vi "Image_Viewer_main.vi"() -> ()   [LabVIEW 2020]
uses:
  #typedef_Program_Data.ctl
  <vilib>/Utility/miscctls.llb/LVBoundsTypeDef.ctl
  <vilib>/event_ctls.llb/eventvkey.ctl
panel:
  out "Program Data":T1
  out "new picture":picture
  out "Multi Listbox":i32(listbox)=-1
  in  "Path":path
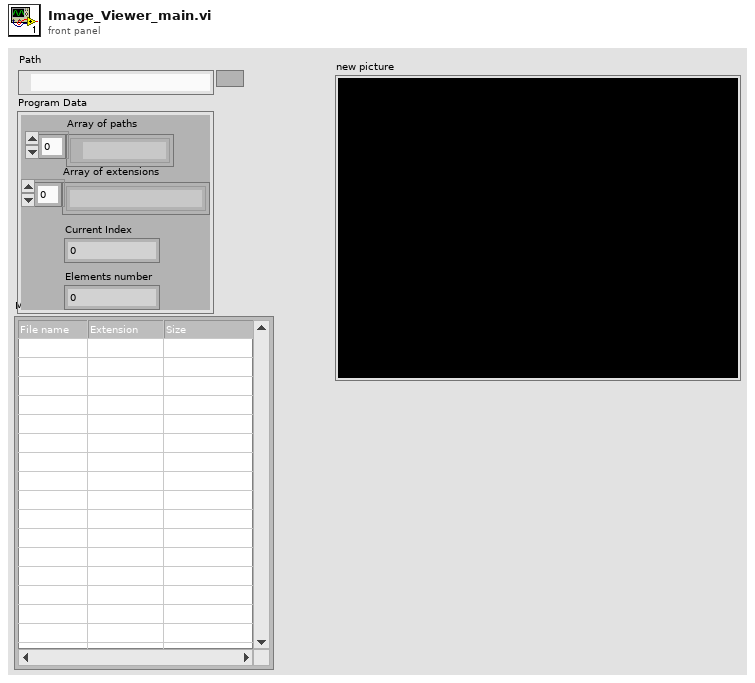
[diagram p1: front panel]
types:
  T1 = typedef "#typedef_Program_Data.ctl" = cluster{"Array of extensions ":string[], "Array of paths":path[], "Current Index":i32, "Elements number":i32}
  T2 = typedef "LVBoundsTypeDef.ctl" = cluster{"Width":u32, "Height":u32}
  T3 = typedef "imagedata.ctl" = cluster{"image type":i32, "image depth":i32, "image":u8[], "mask":u8[], "colors":u32[], "Rectangle":cluster{"left":i16, "top":i16, "right":i16, "bottom":i16}}
  T4 = typedef "eventvkey.ctl" = enum16{"ASCII", "Enter", "Return", "Shift", "Ctrl", "Alt", "Cmd", "Opt", "Caps", "NumLock", "Clear", "Break", "Up", "Down", "Left", "Right", "Insert", "Delete", "Home", "End", "PageUp", "PageDown", "Escape", "Help", "Pause", "ScrollLock", "F1", "F2", "F3", "F4", "F5", "F6", "F7", "F8", "F9", "F10", "F11", "F12", "F13", "F14", "F15", "F16", "F17", "F18", "F19", "F20", "F21", "F22", "F23", "F24", "Play", "VolumeUp", "VolumeDown", "Mute", "Two Byte Char"}
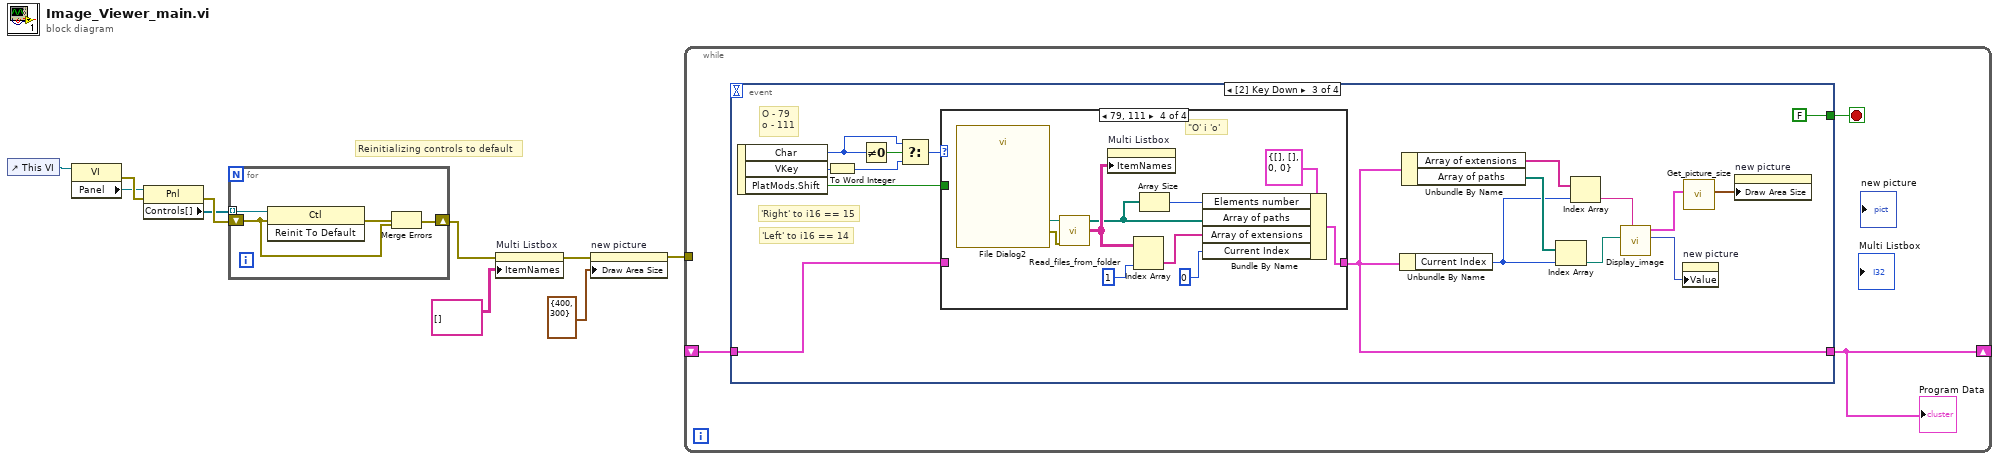
[diagram p0: block diagram]
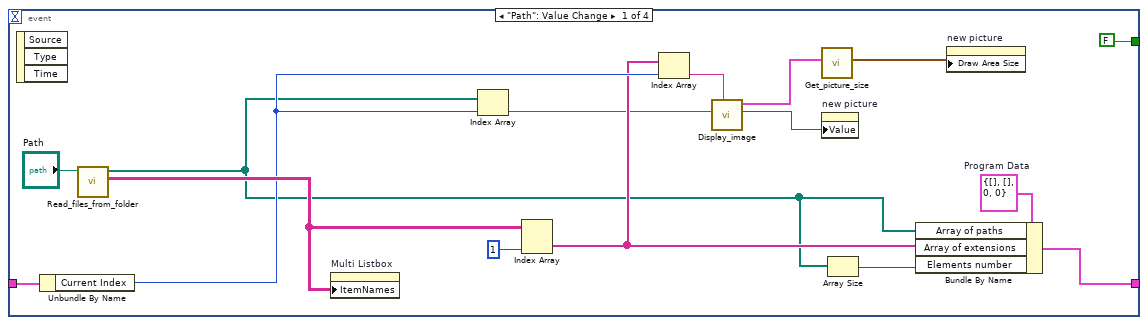
[diagram p2: hidden frame]
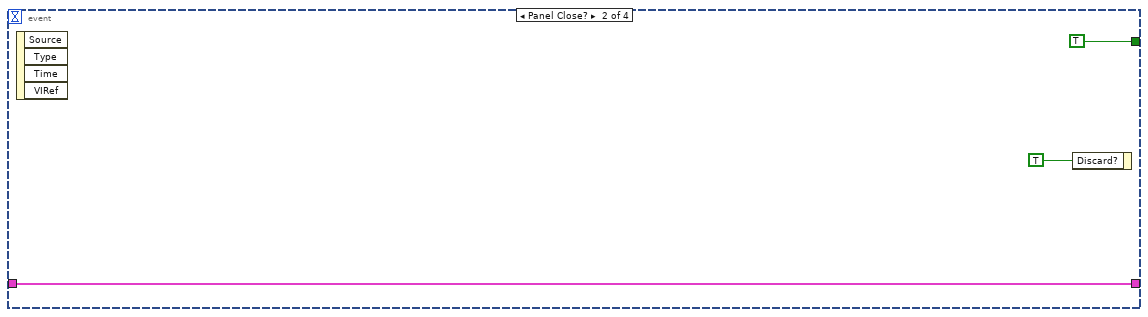
[diagram p3: hidden frame]
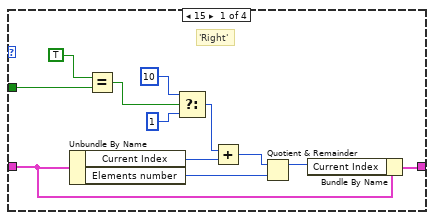
[diagram p4: hidden frame]
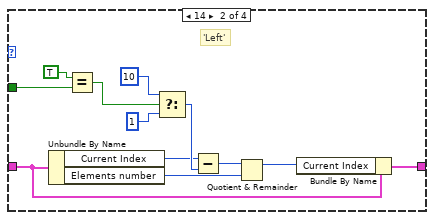
[diagram p5: hidden frame]
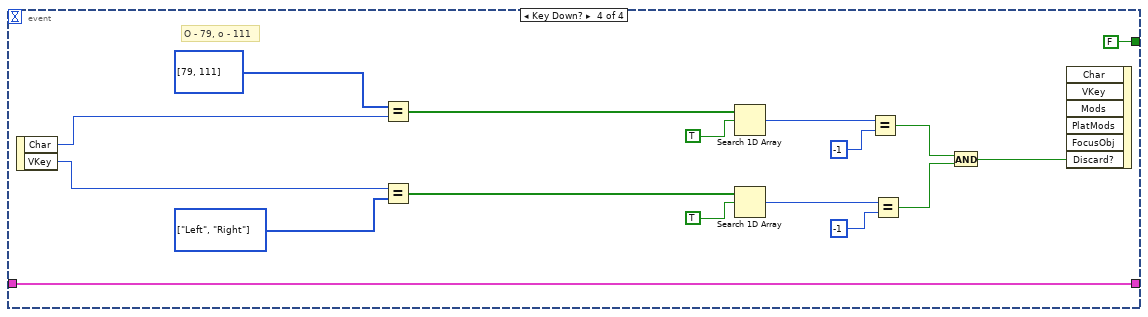
[diagram p7: hidden frame]
diagram:
  # "Reinitializing controls to default"
  n1 = control-ref of="This VI"() -> (w5:refnum<vi>)
  n2 = property class="VI"(reference=w5) -> (error out=w8:errorcluster, "Panel"=w6:refnum<vi>)  [unwired: 1 in, 1 out]
  n3 = property class="Pnl"(reference=w6, error in=w8) -> (error out=w9:errorcluster, "Controls[]"=w7:refnum<vi>[])  [unwired: 1 out]
  n4 = for {
    tunnel: w7 -> [w14] mode=indexing
    shift-right: [w13] -> w2
    shift-left: w9 -> [w12]
    n5 = invoke class="Ctl" method="Reinit To Default"(reference=w14, error in=w12) -> (error out=w11:errorcluster)  [unwired: 1 in, 2 out]
    n6 = Merge Errors(w11, w12) -> (w13:errorcluster)
  }
  n7 = property on="Multi Listbox" class="MCListbox (strict)"(error in=w2, "ItemNames"=string[][] [] ("Item Names")) -> (error out=w1:errorcluster)  [unwired: 1 in, 1 out]
  n8 = property on="new picture" class="Pict"(error in=w1, "Draw Area Size"=T2 {"Width"=400, "Height"=300}) -> (error out=w10:errorcluster)  [unwired: 1 in, 1 out]
  n9 = while {
    shift-right: [w16] -> _
    shift-left: _ -> [w17]
    tunnel: w10 -> [_]
    stop <- w15 stop-if-true
    n10 = event shown="[2] Key Down" {
      selector: _ -> [_ _ _ _]
      dyn-events: _ -> [_ _ _ _]
      timeout: _ -> [_ _ _ _]
      tunnel: w17 -> [w29 w34 w40 w99]
      tunnel: [w18 w34 w38 w99] -> w16
      tunnel: [FALSE TRUE FALSE FALSE] -> w15
      event "Path": Value Change {
        w31 = T1 {"Array of extensions "=[], "Array of paths"=[], "Current Index"=0, "Elements number"=0}  # Program Data
        n11 = event-data() -> ()  [unwired: 1 in, 3 out]
        n12 = Unbundle By Name(w29) -> ("Current Index"=w28:i32)
        n13 = call "Read_files_from_folder.vi"("Path"="Path") -> ("Array of strings (file name, extension, size (in bytes))"=w33:string[][], "File Path"=w20:path[])  [unwired: 8 in, 1 out]
        n14 = property on="Multi Listbox" class="MCListbox (strict)"("ItemNames"=w33) -> ()  [unwired: 2 in, 2 out]
        n15 = Index Array(array=w20, index=w28) -> (element=w26:path)
        n16 = Index Array(array=w33, index (col)=1 ("disabled index (col)")) -> (element=w27:string[])  [unwired: 1 in]
        n17 = Index Array(array=w27, index=w28) -> (element=w24:string)
        n18 = call "Display_image.vi"("lowercase file extension"=w24, "path file"=w26) -> ("picture"=w25:picture, "image data"=w22:T3)  [unwired: 7 in, 1 out]
        n19 = call "Get_picture_size.vi"("image data"=w22) -> ("Draw Area Size"=w21:T2)  [unwired: 9 in, 1 out]
        n20 = property on="new picture" class="Pict"("Value"=w25) -> ()  [unwired: 2 in, 2 out]
        n21 = Array Size(array=w20) -> (size(s)=w19:i32)
        n22 = Bundle By Name(cluster=w31, "Array of paths"=w20, "Array of extensions"=w27, "Elements number"=w19) -> (w18:T1)
        n23 = property on="new picture" class="Pict"("Draw Area Size"=w21) -> ()  [unwired: 2 in, 2 out]
      }
      event Panel Close? {
        n24 = event-data() -> ()  [unwired: 1 in, 4 out]
        n25 = event-data("Discard?"=TRUE) -> ()  [unwired: 1 in, 1 out]
      }
      event Key Down {
        # "O - 79\no - 111"
        # "'Left' to i16 == 14"
        # "'Right' to i16 == 15"
        n26 = event-data() -> ("Char"=w44:i16, "VKey"=w43:T4, "PlatMods.Shift"=w39:bool)  [unwired: 1 in]
        n27 = To Word Integer(number=w43) -> (16bit integer=w42:i16)
        n28 = Not Equal To 0?(x=w44) -> (x != 0?=w45:bool)
        n29 = Select(t=w44, s=w45, f=w42) -> (s? t:f=w41:i16)
        n30 = case shown="79, 111" w41 {
          tunnel: [w55 w68 w78 w79] -> w38
          tunnel: w39 -> [w58 w69 _ _]
          tunnel: w40 -> [w54 w67 w78 _]
          frame 15 {
            # "'Right'"
            n31 = Unbundle By Name(w54) -> ("Current Index"=w61:i32, "Elements number"=w60:i32)
            n32 = Equal?(x=TRUE ("y"), y=w58) -> (x = y?=w65:bool)
            n33 = Select(t=10, s=w65, f=1) -> (s? t:f=w63:i32)
            n34 = Add(x=w63, y=w61) -> (x+y=w59:i32)
            n35 = Quotient & Remainder(x=w59, y=w60) -> (x-y*floor(x/y)=w56:i32)  [unwired: 1 out]
            n36 = Bundle By Name(cluster=w54, "Current Index"=w56) -> (w55:T1)
          }
          frame 14 {
            # "'Left'"
            n37 = Unbundle By Name(w67) -> ("Current Index"=w73:i32, "Elements number"=w71:i32)
            n38 = Equal?(x=TRUE ("y"), y=w69) -> (x = y?=w77:bool)
            n39 = Select(t=10, s=w77, f=1) -> (s? t:f=w74:i32)
            n40 = Subtract(x=w73, y=w74) -> (x-y=w72:i32)
            n41 = Quotient & Remainder(x=w72, y=w71) -> (x-y*floor(x/y)=w66:i32)  [unwired: 1 out]
            n42 = Bundle By Name(cluster=w67, "Current Index"=w66) -> (w68:T1)
          }
          frame Default {
          }
          frame 79, 111 {
            # "\"O' i 'o'"
            n43 = call "File Dialog2"() -> ("selected path"=w88:path, "error out"=w87:errorcluster)  [unwired: 12 in, 2 out]
            n44 = call "Read_files_from_folder.vi"("error in (no error)"=w87, "Path"=w88) -> ("Array of strings (file name, extension, size (in bytes))"=w85:string[][], "File Path"=w81:path[])  [unwired: 7 in, 1 out]
            n45 = property on="Multi Listbox" class="MCListbox (strict)"("ItemNames"=w85) -> ()  [unwired: 2 in, 2 out]
            n46 = Index Array(array=w85, index (col)=1 ("disabled index (col)")) -> (element=w83:string[])  [unwired: 1 in]
            n47 = Array Size(array=w81) -> (size(s)=w82:i32)
            n48 = Bundle By Name(cluster=T1 {"Array of extensions "=[], "Array of paths"=[], "Current Index"=0, "Elements number"=0} ("Program Data"), "Elements number"=w82, "Array of paths"=w81, "Array of extensions"=w83, "Current Index"=0) -> (w79:T1)
          }
        }
        n49 = Unbundle By Name(w38) -> ("Current Index"=w37:i32)
        n50 = Unbundle By Name(w38) -> ("Array of extensions"=w53:string[], "Array of paths"=w52:path[])
        n51 = Index Array(array=w52, index=w37) -> (element=w50:path)
        n52 = Index Array(array=w53, index=w37) -> (element=w51:string)
        n53 = call "Display_image.vi"("lowercase file extension"=w51, "path file"=w50) -> ("picture"=w49:picture, "image data"=w47:T3)  [unwired: 7 in, 1 out]
        n54 = property on="new picture" class="Pict"("Value"=w49) -> ()  [unwired: 2 in, 2 out]
        n55 = call "Get_picture_size.vi"("image data"=w47) -> ("Draw Area Size"=w46:T2)  [unwired: 9 in, 1 out]
        n56 = property on="new picture" class="Pict"("Draw Area Size"=w46) -> ()  [unwired: 2 in, 2 out]
      }
      event Key Down? {
        w104 = T4[] [enum."Left", enum."Right"] items=["ASCII", "Enter", "Return", "Shift", "Ctrl", "Alt", "Cmd", "Opt", "Caps", "NumLock", "Clear", "Break", "Up", "Down", "Left", "Right", "Insert", "Delete", "Home", "End", "PageUp", "PageDown", "Escape", "Help", "Pause", "ScrollLock", "F1", "F2", "F3", "F4", "F5", "F6", "F7", "F8", "F9", "F10", "F11", "F12", "F13", "F14", "F15", "F16", "F17", "F18", "F19", "F20", "F21", "F22", "F23", "F24", "Play", "VolumeUp", "VolumeDown", "Mute", "Two Byte Char"]
        # "O - 79, o - 111"
        n57 = event-data() -> ("Char"=w89:i16, "VKey"=w105:T4)  [unwired: 1 in]
        n58 = Equal?(x=i16[] [79, 111], y=w89) -> (x = y?=w97:bool[])
        n59 = Equal?(x=w105, y=w104) -> (x = y?=w103:bool[])
        n60 = Search 1D Array(1D array=w97, element=TRUE) -> (index of element=w95:i32)  [unwired: 1 in]
        n61 = Search 1D Array(1D array=w103, element=TRUE) -> (index of element=w101:i32)  [unwired: 1 in]
        n62 = Equal?(x=w95, y=-1) -> (x = y?=w93:bool)
        n63 = Equal?(x=w101, y=-1) -> (x = y?=w92:bool)
        n64 = And(x=w93, y=w92) -> (x .and. y?=w91:bool)
        n65 = event-data("Discard?"=w91) -> ()  [unwired: 6 in, 1 out]
      }
    }
    "Program Data" <- w16
  }
